vi "Write Sensor Servo Angle.vi"(8 "error in (no error)":errorcluster, 10 "ccw servo angle (rad)":dbl, 11 "starter kit host in":refnum<class "NI_Robotics_Starter Kit Host.lvclass">) -> (0 "error out":errorcluster, 3 "starter kit host out":refnum<class "NI_Robotics_Starter Kit Host.lvclass">)   [LabVIEW 2017, in "NI_Robotics_Starter Kit Host.lvclass"]
doc: "<B>Owning Palette:</B> Starter Kit 1.0 VIs, Starter Kit 2.0 VIs\n\nWrites an angle to the servo on which the distance sensor is mounted to turn the servo to that angle. Note that the servo angle is different from the sensor angle if the servo and the sensor are not aligned."
uses:
  <vilib>/robotics/Starter Kit/Host Interface/NI_Robotics_Starter Kit Host.lvclass
  <vilib>/robotics/Starter Kit/Host Interface/NI_Robotics_Starter Kit Host.lvclass/NI_Robotics_Starter Kit Host.ctl
  <vilib>/robotics/Starter Kit/Servo Motor/NI_Robotics_Starter Kit Servo Motor.lvclass
  <vilib>/robotics/Utilities/NI_Robotics Utilities.lvlib
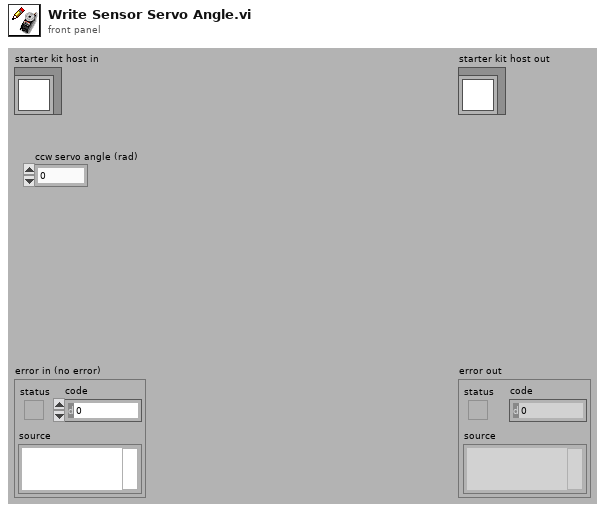
[diagram p1: front panel]
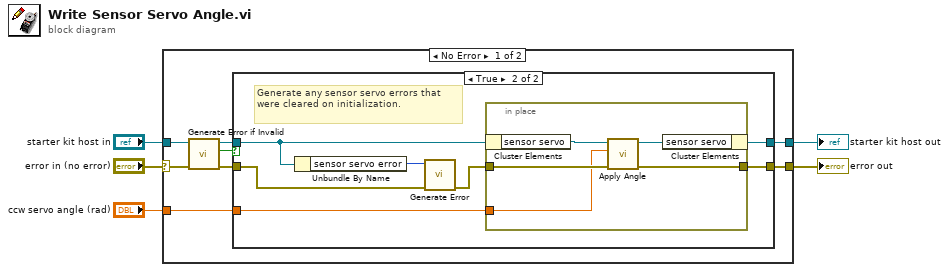
[diagram p0: block diagram]
diagram:
  n1 = case shown="No Error" "error in (no error)" {
    selector: "error in (no error)" -> [w8 w29]
    tunnel: [w12 w29] -> w4
    tunnel: [w13 w28] -> w2
    tunnel: "starter kit host in" -> [w10 w28]
    tunnel: "ccw servo angle (rad)" -> [w11 _]
    frame No Error {
      n2 = call <vilib>:"Generate Error if Invalid.vi"("error in (no error)"=w8, "starter kit host in"=w10) -> ("error out"=w7:errorcluster, "valid?"=w6:bool, "starter kit host out"=w9:refnum<class "NI_Robotics_Starter Kit Host.lvclass">)  [unwired: 7 in]
      n3 = case shown="True" w6 {
        tunnel: [w15 w22] -> w13
        tunnel: [w14 w21] -> w12
        tunnel: w11 -> [_ w20]
        tunnel: w9 -> [w15 w18]
        tunnel: w7 -> [w14 w17]
        frame False {
        }
        frame True {
          # "Generate any sensor servo errors that were cleared on initialization."
          n4 = Unbundle By Name(w18) -> ("sensor servo error"=w19:i32)
          n5 = call <vilib>:"Generate Error.vi"("error in (no error)"=w17, "code"=w19) -> ("error out"=w16:errorcluster)  [unwired: 9 in]
          n6 = in-place {
            in-place-border: w16 -> [w25]
            in-place-border: [w24] -> w21
            in-place-border: w20 -> [w23]
            n7 = in-place-cluster #1(w18) -> ("sensor servo"=w27:refnum<class "NI_Robotics_Starter Kit Servo Motor.lvclass">)
            n8 = call-dynamic "Apply Angle.vi"("error in (no error)"=w25, "ccw servo angle (rad)"=w23, "servo motor in"=w27) -> ("error out"=w24:errorcluster, "servo motor out"=w26:refnum<class "NI_Robotics_Starter Kit Servo Motor.lvclass">)  [unwired: 7 in]
            n9 = in-place-cluster #1("sensor servo"=w26) -> (w22:refnum<class "NI_Robotics_Starter Kit Host.lvclass">)
          }
        }
      }
    }
    frame Error {
    }
  }
  "error out" <- w4
  "starter kit host out" <- w2
